vi "UpdateScrollbarBeforeKeyEvent.vi"(8 "error in (no error)":errorcluster, 10 "VKey":T2, 11 "control refs 2":T1) -> (0 "error out":errorcluster, 2 "LoadBuffer?":bool, 3 "DiscardEvent?":bool)   [LabVIEW 2020]
uses:
  <vilib>/event_ctls.llb/eventvkey.ctl
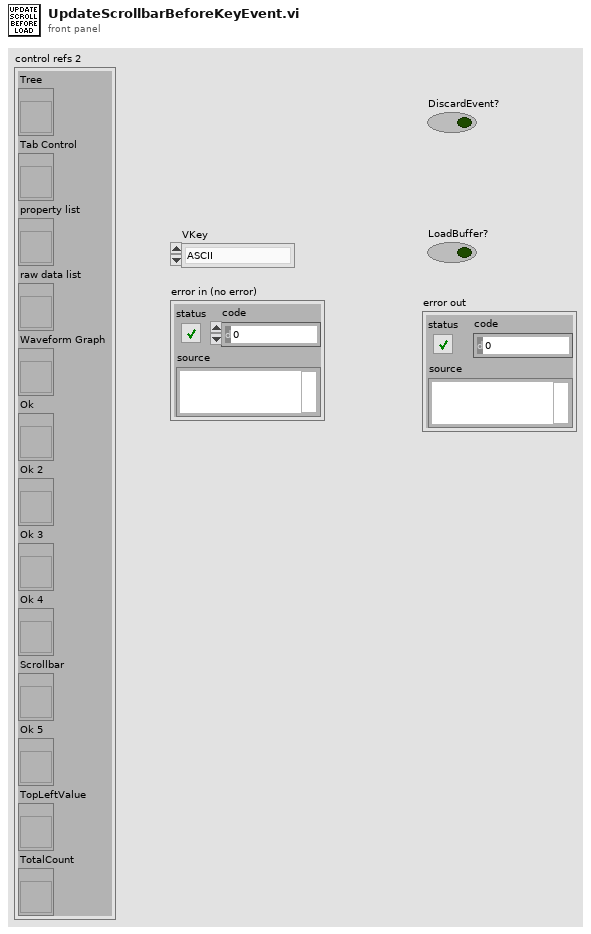
[diagram p1: front panel]
types:
  T1 = cluster{"Tree":refnum<vi>, "Tab Control":refnum<vi>, "property list":refnum<vi>, "raw data list":refnum<vi>, "Waveform Graph":refnum<vi>, "Ok":refnum<vi>, "Ok 2":refnum<vi>, "Ok 3":refnum<vi>, "Ok 4":refnum<vi>, "Scrollbar":refnum<vi>, "Ok 5":refnum<vi>, "TopLeftValue":refnum<vi>, "TotalCount":refnum<vi>}
  T2 = typedef "eventvkey.ctl" = enum16{"ASCII", "Enter", "Return", "Shift", "Ctrl", "Alt", "Cmd", "Opt", "Caps", "NumLock", "Clear", "Break", "Up", "Down", "Left", "Right", "Insert", "Delete", "Home", "End", "PageUp", "PageDown", "Escape", "Help", "Pause", "ScrollLock", "F1", "F2", "F3", "F4", "F5", "F6", "F7", "F8", "F9", "F10", "F11", "F12", "F13", "F14", "F15", "F16", "F17", "F18", "F19", "F20", "F21", "F22", "F23", "F24", "Play", "VolumeUp", "VolumeDown", "Mute", "Two Byte Char"}
  T3 = typedef "LVRowAndColumnUnsignedTypeDef.ctl" = cluster{"Row":u32, "Column":u32}
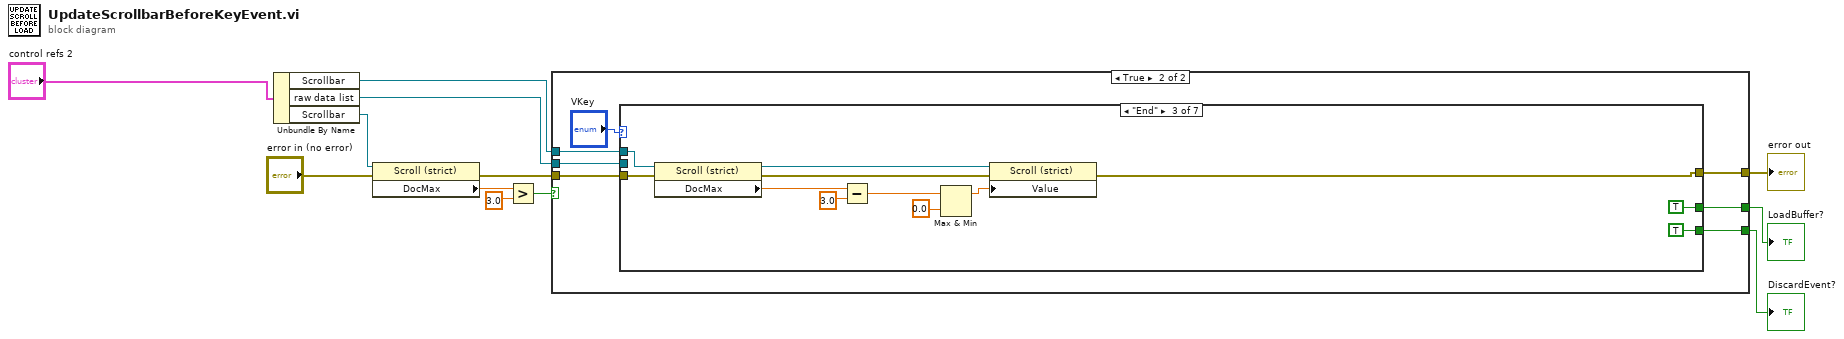
[diagram p0: block diagram]
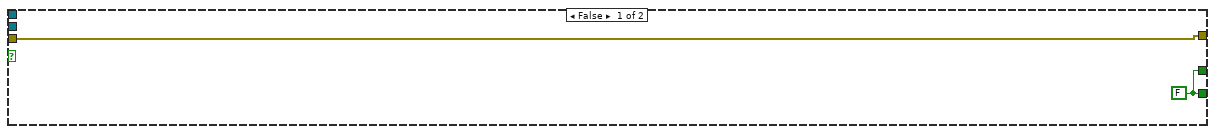
[diagram p2: hidden frame]
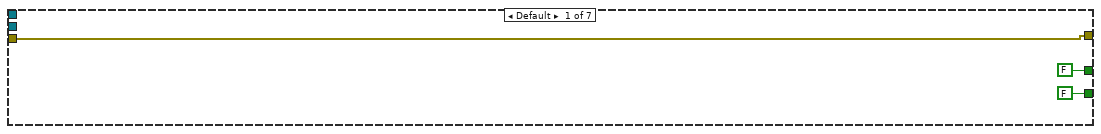
[diagram p3: hidden frame]
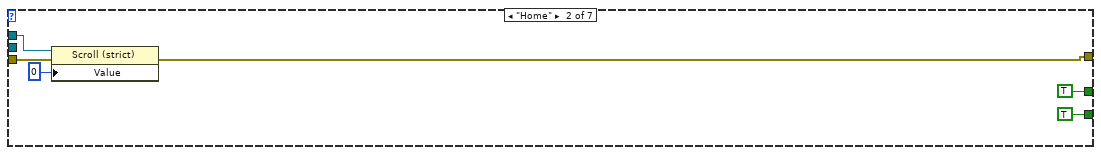
[diagram p4: hidden frame]
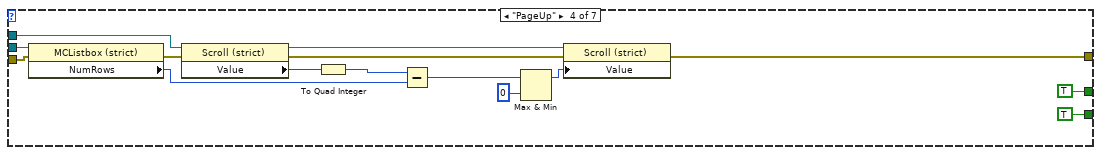
[diagram p5: hidden frame]
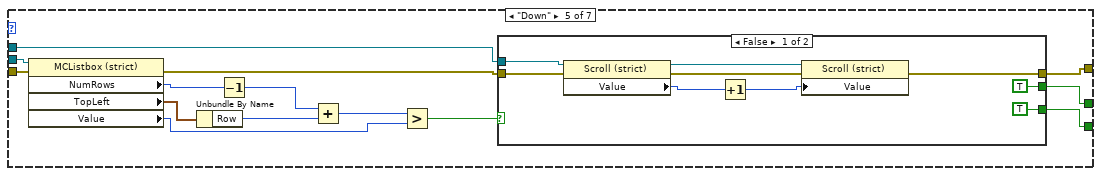
[diagram p6: hidden frame]
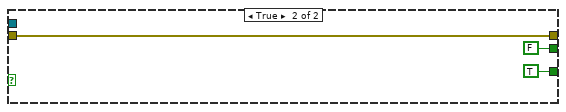
[diagram p7: hidden frame]
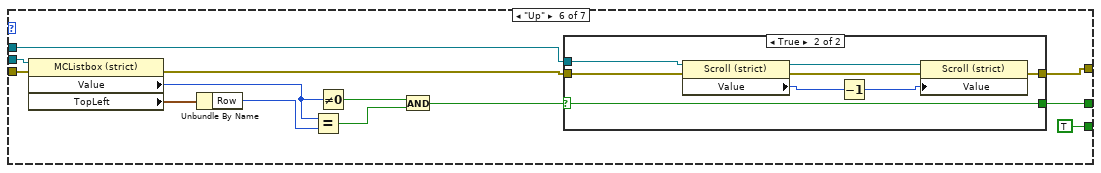
[diagram p8: hidden frame]
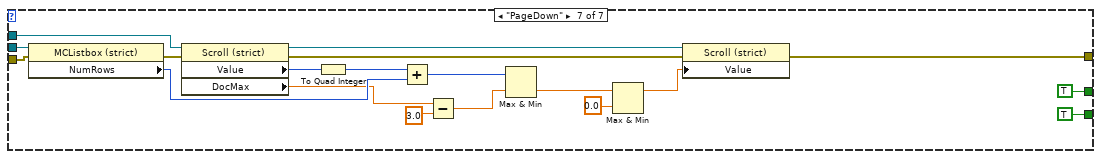
[diagram p10: hidden frame]
diagram:
  n1 = Unbundle By Name("control refs 2") -> ("Scrollbar"=w9:refnum<vi>, "raw data list"=w8:refnum<vi>, "Scrollbar"=w5:refnum<vi>)
  n2 = property on="Property Node" class="Scroll (strict)"(reference=w5, error in="error in (no error)") -> (error out=w6:errorcluster, "DocMax"=w3:dbl)  [unwired: 1 out]
  n3 = Greater?(x=w3, y=3.0) -> (0:w2:bool)
  n4 = case shown="True" w2 {
    tunnel: [w14 w21] -> w12
    tunnel: [w14 w20] -> w11
    tunnel: [w13 w18] -> w10
    tunnel: w9 -> [_ w17]
    tunnel: w8 -> [_ w16]
    tunnel: w6 -> [w13 w15]
    frame False {
      w14 = FALSE
    }
    frame True {
      n5 = case shown="\"End\"" "VKey" {
        tunnel: [FALSE TRUE TRUE TRUE w71 TRUE TRUE] -> w20
        tunnel: w15 -> [w23 w29 w41 w52 w58 w96 w121]
        tunnel: [w23 w27 w35 w55 w70 w86 w123] -> w18
        tunnel: [FALSE TRUE TRUE TRUE w69 w85 TRUE] -> w21
        tunnel: w17 -> [_ w25 w32 w44 w67 w87 w108]
        tunnel: w16 -> [_ _ _ w45 w68 w95 w109]
        frame Default {
        }
        frame "Home" {
          n6 = property on="Property Node" class="Scroll (strict)"(reference=w25, error in=w29, "Value"=u64 0 ("Scrollbar")) -> (error out=w27:errorcluster)  [unwired: 1 out]
        }
        frame "End" {
          n7 = property on="Property Node" class="Scroll (strict)"(reference=w32, error in=w41) -> (reference out=w31:refnum<vi>, error out=w36:errorcluster, "DocMax"=w40:dbl)
          n8 = Subtract(x=w40, y=3.0 ("Raw data values")) -> (x-y=w38:dbl)
          n9 = Max & Min(x=w38, y=0.0) -> (max(x,y)=w34:dbl)  [unwired: 1 out]
          n10 = property on="Property Node" class="Scroll (strict)"(reference=w31, error in=w36, "Value"=w34) -> (error out=w35:errorcluster)  [unwired: 1 out]
        }
        frame "PageUp" {
          n11 = property on="Property Node" class="MCListbox (strict)"(reference=w45, error in=w52) -> (error out=w51:errorcluster, "NumRows"=w50:u32)  [unwired: 1 out]
          n12 = property on="Property Node" class="Scroll (strict)"(reference=w44, error in=w51) -> (reference out=w43:refnum<vi>, error out=w48:errorcluster, "Value"=w47:u64)
          n13 = To Quad Integer(1:w47) -> (0:w46:i64)
          n14 = Subtract(x=w46, y=w50) -> (x-y=w56:i64)
          n15 = Max & Min(x=w56, y=i64 0) -> (max(x,y)=w54:i64)  [unwired: 1 out]
          n16 = property on="Property Node" class="Scroll (strict)"(reference=w43, error in=w48, "Value"=w54) -> (error out=w55:errorcluster)  [unwired: 1 out]
        }
        frame "Down" {
          n17 = property on="Property Node" class="MCListbox (strict)"(reference=w68, error in=w58) -> (error out=w59:errorcluster, "NumRows"=w65:u32, "TopLeft"=w66:T3, "Value"=w61:i32)  [unwired: 1 out]
          n18 = Unbundle By Name(w66) -> ("Row"=w63:u32)
          n19 = Decrement(x=w65) -> (x-1=w64:u32)
          n20 = Add(x=w64, y=w63) -> (x+y=w62:u32)
          n21 = Greater?(x=w62, y=w61) -> (0:w60:bool)
          n22 = case shown="False" w60 {
            tunnel: [TRUE TRUE] -> w71
            tunnel: [TRUE FALSE] -> w69
            tunnel: w59 -> [w80 w81]
            tunnel: [w74 w81] -> w70
            tunnel: w67 -> [w79 _]
            frame False {
              n23 = property on="Property Node" class="Scroll (strict)"(reference=w79, error in=w80) -> (reference out=w76:refnum<vi>, error out=w75:errorcluster, "Value"=w78:u64)
              n24 = Increment(x=w78) -> (x+1=w77:u64)
              n25 = property on="Property Node" class="Scroll (strict)"(reference=w76, error in=w75, "Value"=w77) -> (error out=w74:errorcluster)  [unwired: 1 out]
            }
            frame True {
            }
          }
        }
        frame "Up" {
          n26 = property on="Property Node" class="MCListbox (strict)"(reference=w95, error in=w96) -> (error out=w88:errorcluster, "Value"=w92:i32, "TopLeft"=w94:T3)  [unwired: 1 out]
          n27 = Unbundle By Name(w94) -> ("Row"=w93:u32)
          n28 = Equal?(x=w92, y=w93) -> (x = y?=w91:bool)
          n29 = Not Equal To 0?(x=w92) -> (x != 0?=w90:bool)
          n30 = And(x=w90, y=w91) -> (x .and. y?=w89:bool)
          n31 = case shown="True" w89 {
            selector: w89 -> [w97 w99]
            tunnel: w88 -> [w98 w102]
            tunnel: w87 -> [_ w101]
            tunnel: [w98 w100] -> w86
            tunnel: [w97 w99] -> w85
            frame False {
            }
            frame True {
              n32 = property on="Property Node" class="Scroll (strict)"(reference=w101, error in=w102) -> (reference out=w104:refnum<vi>, error out=w103:errorcluster, "Value"=w106:u64)
              n33 = Decrement(x=w106) -> (x-1=w105:u64)
              n34 = property on="Property Node" class="Scroll (strict)"(reference=w104, error in=w103, "Value"=w105) -> (error out=w100:errorcluster)  [unwired: 1 out]
            }
          }
        }
        frame "PageDown" {
          n35 = property on="Property Node" class="MCListbox (strict)"(reference=w109, error in=w121) -> (error out=w120:errorcluster, "NumRows"=w119:u32)  [unwired: 1 out]
          n36 = property on="Property Node" class="Scroll (strict)"(reference=w108, error in=w120) -> (reference out=w107:refnum<vi>, error out=w118:errorcluster, "Value"=w117:u64, "DocMax"=w115:dbl)
          n37 = To Quad Integer(1:w117) -> (0:w116:i64)
          n38 = Add(x=w116, y=w119) -> (x+y=w124:i64)
          n39 = Subtract(x=w115, y=3.0) -> (x-y=w113:dbl)
          n40 = Max & Min(x=w124, y=w113) -> (min(x,y)=w112:dbl)  [unwired: 1 out]
          n41 = Max & Min(x=w112, y=0.0) -> (max(x,y)=w110:dbl)  [unwired: 1 out]
          n42 = property on="Property Node" class="Scroll (strict)"(reference=w107, error in=w118, "Value"=w110) -> (error out=w123:errorcluster)  [unwired: 1 out]
        }
      }
    }
  }
  "LoadBuffer?" <- w12
  "DiscardEvent?" <- w11
  "error out" <- w10
